vi "Display Mode Value.vi"(4 "Display Mode":T1) -> (7 "DisplayMode":u8 format="%.0x")   [LabVIEW 2020, in "CTI-Peripheral.lvlib" / "HD44780 LCD.lvlib"]
uses:
  HD44780 LCD.lvlib
  Display Mode.ctl
  Character LCD/Entry Shift.ctl
  Character LCD/Glyph Entry.ctl
  Character LCD/Char LCD.lvclass
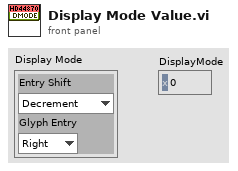
[diagram p1: front panel]
types:
  T1 = typedef "CTI-Peripheral.lvlib/HD44780 LCD.lvlib/Display Mode.ctl" = cluster{"Entry Shift":T2, "Glyph Entry":T3}
  T2 = typedef "CTI-Peripheral.lvlib/Char LCD.lvclass/Entry Shift.ctl" = enum8{"Decrement", "Increment"}
  T3 = typedef "CTI-Peripheral.lvlib/Char LCD.lvclass/Glyph Entry.ctl" = enum8{"Right", "Left"}
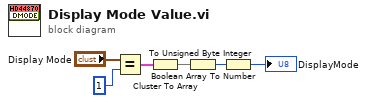
[diagram p0: block diagram]
diagram:
  n1 = Equal?(x="Display Mode", y=1) -> (x = y?=w4:cluster{"Entry Shift":bool, "Glyph Entry":bool})
  n2 = Cluster To Array(cluster=w4) -> (array=w3:bool[])
  n3 = Boolean Array To Number(Boolean array=w3) -> (number=w2:u32)
  n4 = To Unsigned Byte Integer(number=w2) -> (unsigned 8bit integer=→"DisplayMode":u8)
